vi "check_file_size.vi"(3 "error in":errorcluster, 4 "path in":path, 5 "ref in":T1 format="%.0x", 6 "mode (read-only)":T2) -> (0 "error out":errorcluster, 1 "Path":path, 2 "ref out":T1 format="%.0x")   [LabVIEW 2020]
uses:
  <vilib>/addons/h5labview2/file/H5Fmode.ctl
  <vilib>/addons/h5labview2/base/hid_t.ctl
  <vilib>/addons/h5labview2/file/H5F.lvlib
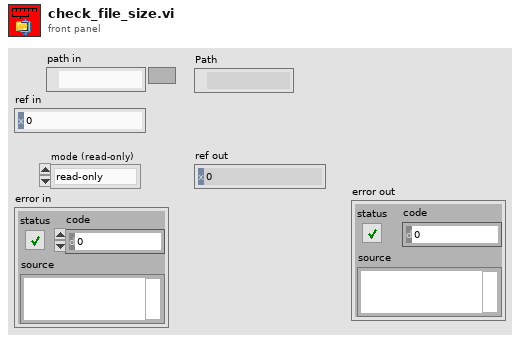
[diagram p1: front panel]
types:
  T1 = typedef "hid_t.ctl" = i64
  T2 = typedef "H5F.lvlib/H5Fmode.ctl" = enum16{"read-only", "read-write", "overwrite", "create new", "open or create"}
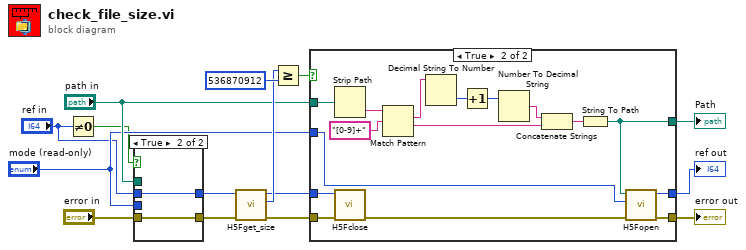
[diagram p0: block diagram]
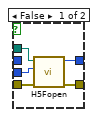
[diagram p2: hidden frame]
diagram:
  n1 = Not Equal To 0?(x="ref in") -> (x != 0?=w4:bool)
  n2 = case shown="True" w4 {
    tunnel: "path in" -> [w20 _]
    tunnel: [w19 w22] -> w10
    tunnel: [w18 w21] -> w1
    tunnel: "mode (read-only)" -> [w17 _]
    tunnel: "ref in" -> [_ w22]
    tunnel: "error in" -> [w16 w21]
    frame False {
      n3 = call <vilib>:"H5Fopen.vi"("error in (no error)"=w16, "mode (read-only)"=w17, "path"=w20) -> ("error out"=w18:errorcluster, "ref out"=w19:T1)  [unwired: 7 in]
    }
    frame True {
    }
  }
  n4 = call <vilib>:"H5Fget_size.vi"("error in (no error)"=w1, "ref in"=w10) -> ("error out"=w7:errorcluster, "size"=w12:u64, "ref out"=w8:T1)  [unwired: 7 in]
  n5 = Greater Or Equal?(x=w12, y=i64 536870912) -> (x >= y?=w14:bool)
  n6 = case shown="True" w14 {
    tunnel: [w25 w29] -> w15
    tunnel: "path in" -> [w25 w34]
    tunnel: [w23 w28] -> w9
    tunnel: w8 -> [w23 w32]
    tunnel: w7 -> [w24 w31]
    tunnel: "mode (read-only)" -> [_ w27]
    tunnel: [w24 w26] -> w5
    frame False {
    }
    frame True {
      n7 = Strip Path(path=w34) -> (name=w33:string)  [unwired: 1 out]
      n8 = call <vilib>:"H5Fclose.vi"("error in (no error)"=w31, "ref"=w32) -> ("error out"=w30:errorcluster)  [unwired: 9 in]
      n9 = Match Pattern(string=w33, regular expression="[0-9]+") -> (match substring=w36:string, after substring=w40:string)  [unwired: 1 in, 2 out]
      n10 = Decimal String To Number(string=w36) -> (number=w39:i32)  [unwired: 2 in, 1 out]
      n11 = Increment(x=w39) -> (x+1=w37:i32)
      n12 = Number To Decimal String(number=w37) -> (decimal integer string=w38:string)  [unwired: 1 in]
      n13 = Concatenate Strings(w38, w40) -> (w35:string)
      n14 = String To Path(string=w35) -> (path=w29:path)
      n15 = call <vilib>:"H5Fopen.vi"("error in (no error)"=w30, "mode (read-only)"=w27, "path"=w29) -> ("error out"=w26:errorcluster, "ref out"=w28:T1)  [unwired: 7 in]
    }
  }
  "Path" <- w15
  "ref out" <- w9
  "error out" <- w5
